vi "hmp4000 Configure General Output State.vi"(8 "error in (no error)":errorcluster, 9 "Output State (Off)":bool, 11 "VISA resource name":refnum<visa-resource-name>) -> (0 "error out":errorcluster, 3 "VISA resource name out":refnum<visa-resource-name>)   [LabVIEW 2022 SP3]
doc: "Turning on / off all previous selected channels simultaneously.\n\nAttribute:\nHMP4000_ATTR_GENERAL_OUTPUT_STATE\n\nRemote-control command:\nOUTPut:GENeral"
uses:
  Instance           1 38Saved   hmp4000 Configure Output State .vi
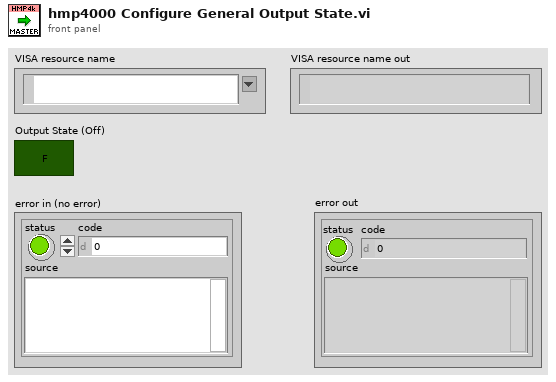
[diagram p1: front panel]
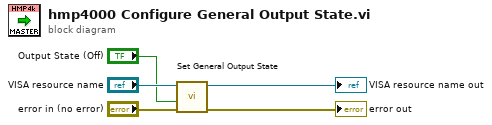
[diagram p0: block diagram]
diagram:
  n1 = call "Set General Output State"("error in (no error)"="error in (no error)", "General Output State (OFF)"="Output State (Off)", "instrument handle"="VISA resource name") -> ("error out"=→"error out":errorcluster, "instrument handle out"=→"VISA resource name out":refnum<visa-resource-name>)  [unwired: 7 in]
